vi "HW_QX_Generate QX Device List Info.vi"(11 "QXModuInfo":T5[](array[typedef])) -> (3 "DevInfo":T1)   [LabVIEW 2016]
uses:
  Ctrls/HardWare Basic Info _ Channel.ctl
  Ctrls/HardWare Basic Info _ Module.ctl
  Ctrls/HardWare Basic Info _ Chassis.ctl
  Ctrls/HardWare Basic Info _ Device.ctl
  QX Module Info.ctl
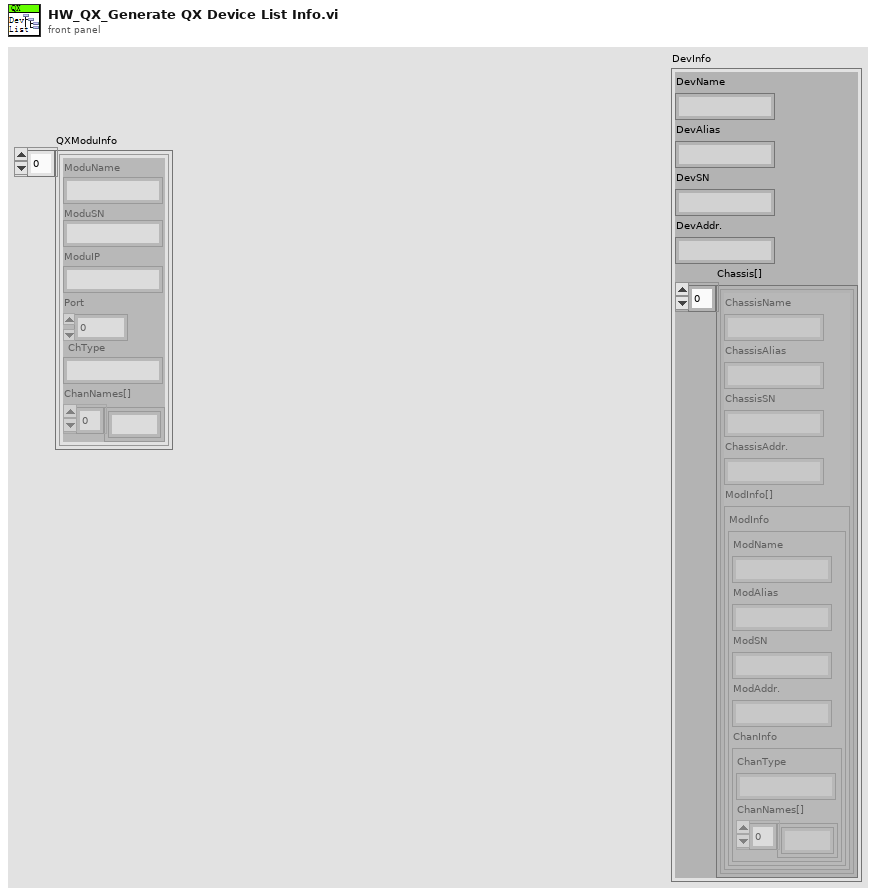
[diagram p1: front panel]
types:
  T1 = typedef "HardWare Basic Info _ Device.ctl" = cluster{"DevName":string, "DevAlias":string, "DevSN":string, "DevAddr.":string, "Chassis[]":T2[]}
  T2 = typedef "HardWare Basic Info _ Chassis.ctl" = cluster{"ChassisName":string, "ChassisAlias":string, "ChassisSN":string, "ChassisAddr.":string, "ModInfo[]":T3[]}
  T3 = typedef "HardWare Basic Info _ Module.ctl" = cluster{"ModName":string, "ModAlias":string, "ModSN":string, "ModAddr.":string, "ChanInfo":T4}
  T4 = typedef "HardWare Basic Info _ Channel.ctl" = cluster{"ChanType":string, "ChanNames[]":string[]}
  T5 = typedef "QX Module Info.ctl" = cluster{"ModuName":string, "ModuSN":string, "ModuIP":string, "Port":i32, "ChType":string, "ChanNames[]":string[]}
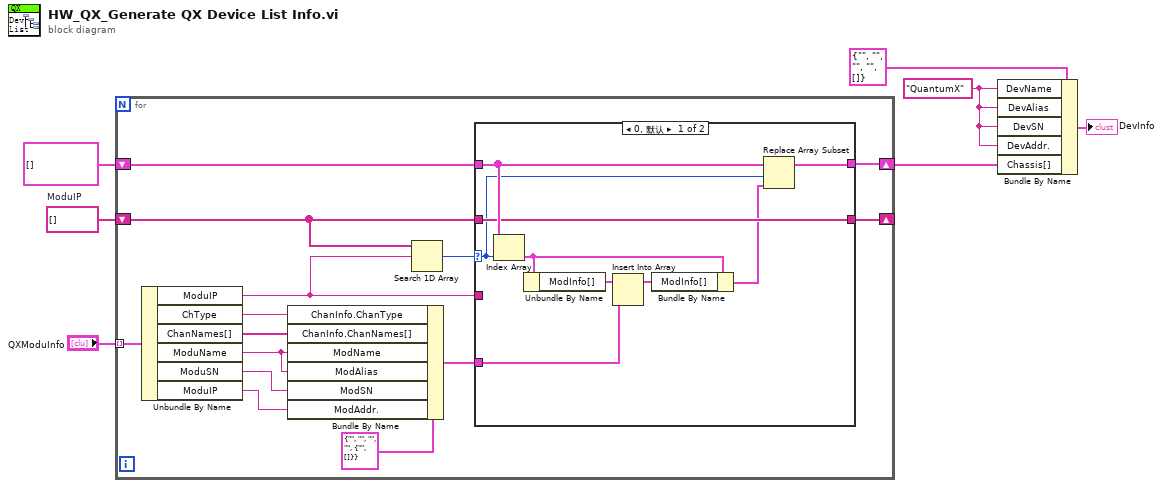
[diagram p0: block diagram]
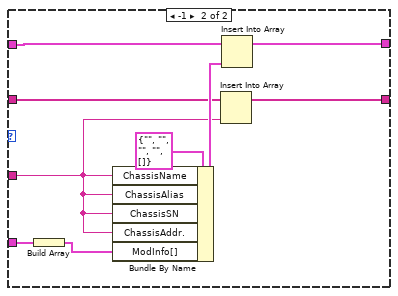
[diagram p2: hidden frame]
diagram:
  w2 = "QuantumX" ("DevName")
  w7 = string[] []  # ModuIP
  n1 = for {
    tunnel: "QXModuInfo" -> [w21] mode=indexing
    shift-right: [w10] -> w3
    shift-left: T2[] [] -> [w19]
    shift-right: [w8] -> _
    shift-left: w7 -> [w9]
    n2 = Unbundle By Name(w21) -> ("ModuIP"=w18:string, "ChType"=w16:string, "ChanNames[]"=w15:string[], "ModuName"=w14:string, "ModuSN"=w13:string, "ModuIP"=w12:string)
    n3 = Bundle By Name(cluster=T3 {"ModName"="", "ModAlias"="", "ModSN"="", "ModAddr."="", "ChanInfo"={"ChanType"="", "ChanNames[]"=[]}} ("ModInfo"), "ChanInfo.ChanType"=w16, "ChanInfo.ChanNames[]"=w15, "ModName"=w14, "ModAlias"=w14, "ModSN"=w13, "ModAddr."=w12) -> (w11:T3)
    n4 = Search 1D Array(1D array=w9, element=w18) -> (index of element=w20:i32)  [unwired: 1 in]
    n5 = case shown="0, 默认" w20 {
      selector: w20 -> [w23 _]
      tunnel: w19 -> [w30 w36]
      tunnel: w18 -> [_ w31]
      tunnel: w11 -> [w27 w38]
      tunnel: [w22 w34] -> w10
      tunnel: w9 -> [w29 w33]
      tunnel: [w29 w32] -> w8
      frame 0, Default {
        n6 = Index Array(array=w30, index=w23) -> (element=w26:T2)
        n7 = Unbundle By Name(w26) -> ("ModInfo[]"=w28:T3[])
        n8 = Insert Into Array(array=w28, new element=w27) -> (w25:T3[])  [unwired: 1 in]
        n9 = Bundle By Name(cluster=w26, "ModInfo[]"=w25) -> (w24:T2)
        n10 = Replace Array Subset(array=w30, new element=w24, index=w23) -> (w22:T2[])
      }
      frame -1 {
        n11 = Build Array(w38) -> (w37:T3[])
        n12 = Bundle By Name(cluster=T2 {"ChassisName"="", "ChassisAlias"="", "ChassisSN"="", "ChassisAddr."="", "ModInfo[]"=[]} ("Chassis"), "ChassisName"=w31, "ChassisAlias"=w31, "ChassisSN"=w31, "ChassisAddr."=w31, "ModInfo[]"=w37) -> (w35:T2)
        n13 = Insert Into Array(array=w33, new element=w31) -> (w32:string[])  [unwired: 1 in]
        n14 = Insert Into Array(array=w36, new element=w35) -> (w34:T2[])  [unwired: 1 in]
      }
    }
  }
  n15 = Bundle By Name(cluster=T1 {"DevName"="", "DevAlias"="", "DevSN"="", "DevAddr."="", "Chassis[]"=[]} ("Device"), "DevName"=w2, "DevAlias"=w2, "DevSN"=w2, "DevAddr."=w2, "Chassis[]"=w3) -> (→"DevInfo":T1)
